vi "CSM - Convert Array to Argument.vi"(2 "DBL":dbl[](array[numeric])) -> (7 "Argument":string)   [LabVIEW 2014, in "Array Parameter Support.lvlib"]
doc: "Convert complex argument(variant) to hex string, which could be safely used as state argument without broking the string queue logic.\n\n<b>Inputs:</b>\n - <b>Variant</b>: Complex data in variant format.\n\n<b>Outputs:</b>\n - <b>HEX String (0-9,A-F)</b>: Hex String, which contains no invisible string following JKISM's rule"
uses:
  Array Parameter Support.lvlib
  _support/Operation-FGV-MassData.ctl
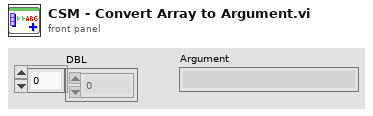
[diagram p1: front panel]
types:
  T1 = typedef "Array Parameter Support.lvlib/Operation-FGV-MassData.ctl" = enum16{"Initialize", "Read", "Write", "Status", "Release"}
  T2 = typedef "Array Parameter Support.lvlib/Def-MassDataOper-Status.ctl" = cluster{"Start":i32, "Size":i32, "Total":i32}
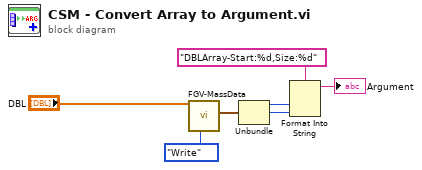
[diagram p0: block diagram]
diagram:
  n1 = call "FGV-MassData.vi"("Operation"=Operation-FGV-MassData."Write", "Data in"="DBL") -> ("Active Write Oper"=w3:T2)  [unwired: 6 in, 3 out]
  n2 = Unbundle(w3) -> ("Start"=w2:i32, "Size"=w1:i32)  [unwired: 1 out]
  n3 = Format Into String(format string="DBLArray-Start:%d,Size:%d", w2, w1) -> (resulting string=→"Argument":string)  [unwired: 2 in, 1 out]
